vi "21-Material Movement.vi"(8 "error in":errorcluster, 11 "Material Movement CEID":u32) -> (0 "error out":errorcluster)   [LabVIEW 2020, in "SECS Scenarios.lvlib" / "Scenarios Class.lvclass"]
uses:
  Scenarios Class.lvclass
  21-Material Movement.ctl
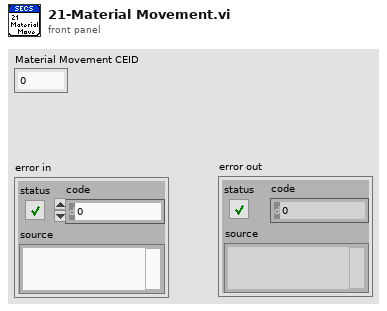
[diagram p1: front panel]
types:
  T1 = typedef "SECS Scenarios.lvlib/Scenarios Class.lvclass/21-Material Movement.ctl" = cluster{"Material Movement CEID":u32}
  T2 = typedef "SECS Scenarios.lvlib/Scenarios Class.lvclass/Request Refnum.ctl" = cluster{"11-Alarm Management":refnum<user-event>, "07-Event Report From Equipment":refnum<user-event>, "14-Process Program Creating Editing or Deleting":refnum<user-event>, "21-Material Movement":refnum<user-event>, "23-Equipment Sends Information to Host":refnum<user-event>, "24-Host Accepts On-Line Request from Equipment":refnum<user-event>, "25-Host Refuses On-Line Request":refnum<user-event>, "29-Equipment Requests Time Value from Host":refnum<user-event>, "33-Update Trace Data":refnum<user-event>}
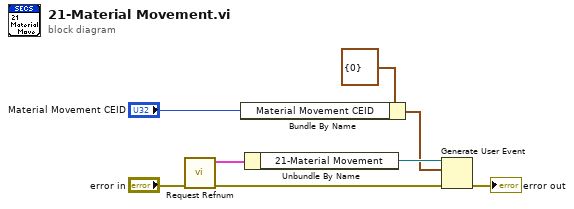
[diagram p0: block diagram]
diagram:
  n1 = call "Request Refnum.vi"("error in"="error in") -> ("error out"=w5:errorcluster, "Request Refnum"=w6:T2)  [unwired: 9 in]
  n2 = Bundle By Name(cluster=T1 {"Material Movement CEID"=0} ("21-Material Movement"), "Material Movement CEID"="Material Movement CEID") -> (w3:T1)
  n3 = Unbundle By Name(w6) -> ("21-Material Movement"=w4:refnum<user-event>)
  n4 = Generate User Event(user event=w4, event data cluster=w3, error in=w5) -> (error out=→"error out":errorcluster)  [unwired: 1 in, 1 out]
